vi "FindLeakMap.vi"(4 "Y":dbl[](array[numeric]), 6 "Y坐标":refnum<vi>, 7 "Z":dbl[](array[numeric]), 9 "X坐标":refnum<vi>, 10 "X":dbl[](array[numeric]), 11 "Z最大值":refnum<vi>) -> ()   [LabVIEW 2014, in "cyy.lvlib" / "LeakageFenXi.lvlib"]
uses:
  LeakageFenXi.lvlib
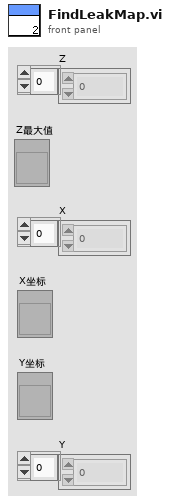
[diagram p1: front panel]
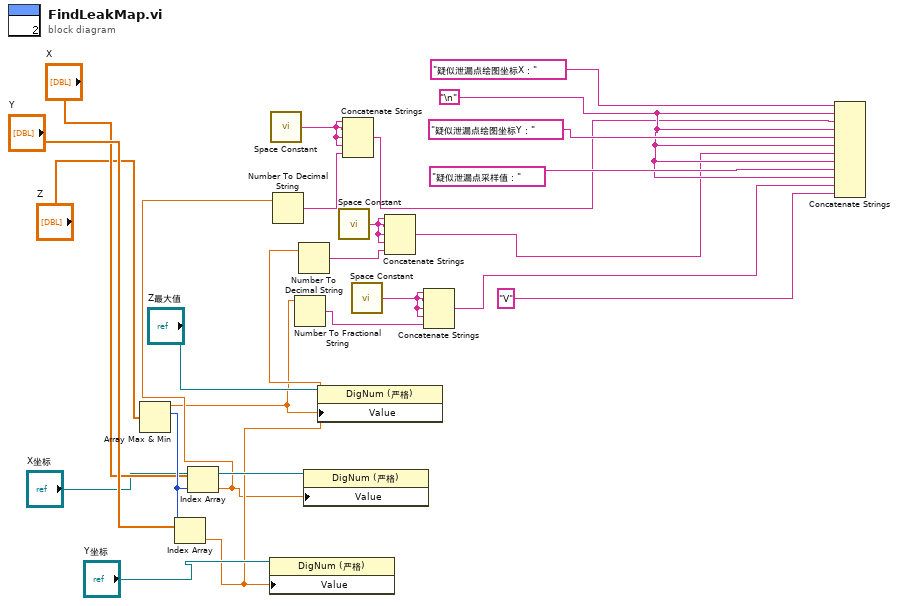
[diagram p0: block diagram]
diagram:
  w14 = "\n"
  n1 = Array Max & Min(array="Z") -> (max value=w1:dbl, max index (indices)=w24:i32)  [unwired: 2 out]
  n2 = Index Array(array="Y", index=w24) -> (element=w3:dbl)
  n3 = Index Array(array="X", index=w24) -> (element=w2:dbl)
  n4 = property class="DigNum (严格)"(reference="Y坐标", "Value"=w3) -> ()  [unwired: 1 in, 2 out]
  n5 = call <vilib>:"Space Constant.vi"() -> ("String"=w12:string)
  n6 = Number To Decimal String(number=w2) -> (decimal integer string=w11:string)  [unwired: 1 in]
  n7 = Number To Fractional String(number=w1) -> (F-format string=w5:string)  [unwired: 3 in]
  n8 = Number To Decimal String(number=w3) -> (decimal integer string=w8:string)  [unwired: 1 in]
  n9 = property class="DigNum (严格)"(reference="X坐标", "Value"=w2) -> ()  [unwired: 1 in, 2 out]
  n10 = property class="DigNum (严格)"(reference="Z最大值", "Value"=w1) -> ()  [unwired: 1 in, 2 out]
  n11 = call <vilib>:"Space Constant.vi"() -> ("String"=w9:string)
  n12 = Concatenate Strings(w12, w12, w12, w12, w11) -> (w10:string)
  n13 = call <vilib>:"Space Constant.vi"() -> ("String"=w6:string)
  n14 = Concatenate Strings(w9, w9, w9, w9, w8) -> (w7:string)
  n15 = Concatenate Strings(w6, w6, w6, w6, w5) -> (w4:string)
  n16 = Concatenate Strings("疑似泄漏点绘图坐标X：", w14, w10, w14, "疑似泄漏点绘图坐标Y：", w14, w7, w14, "疑似泄漏点采样值：", w14, w4, "V") -> ()  [unwired: 1 out]
